vi "Generate.vi"(0 "Snake in":refnum<class "Snake.lvclass">, 1 "Coordinates":T1, 5 "error in (no error)":errorcluster) -> (14 "Snake out":refnum<class "Snake.lvclass">, 19 "error out":errorcluster)   [LabVIEW 2021, in "Snake.lvclass"]
uses:
  Snake.lvclass
  Coordinates.ctl
  Snake.lvclass/Snake.ctl
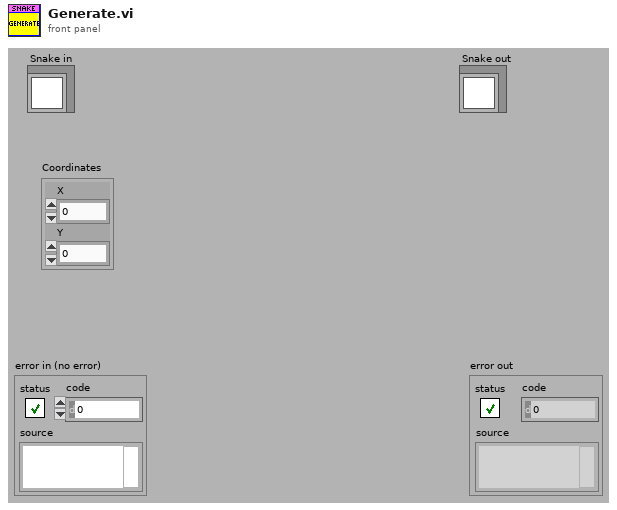
[diagram p1: front panel]
types:
  T1 = typedef "Coordinates.ctl" = cluster{"X":i32, "Y":i32}
  T2 = typedef "Direction.ctl" = enum16{"up", "down", "left", "right"}
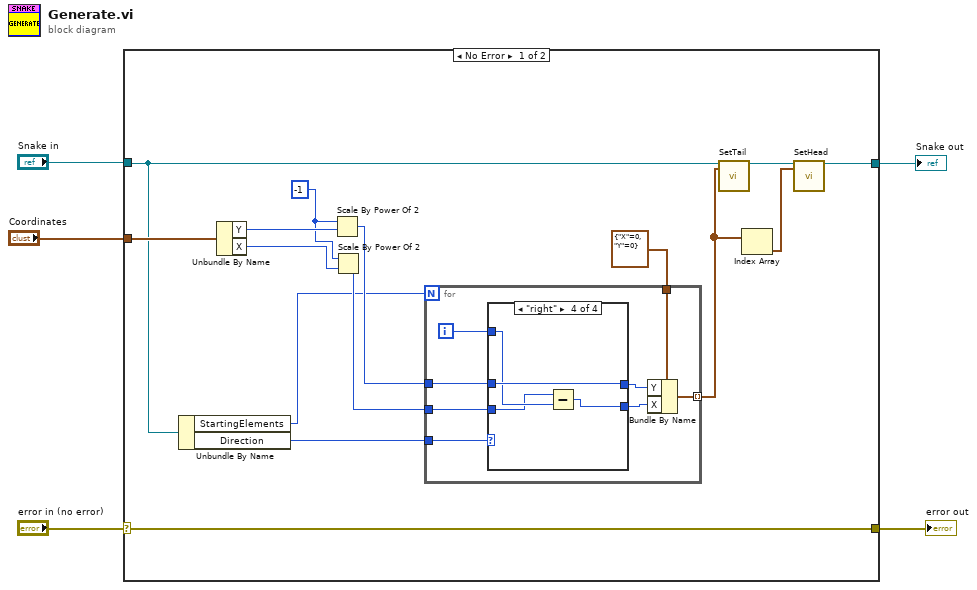
[diagram p0: block diagram]
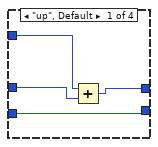
[diagram p2: hidden frame]
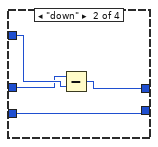
[diagram p3: hidden frame]
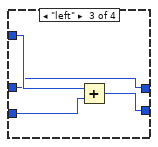
[diagram p4: hidden frame]
diagram:
  n1 = case shown="No Error" "error in (no error)" {
    selector: "error in (no error)" -> [w20 w46]
    tunnel: [w20 w46] -> w4
    tunnel: [w9 w45] -> w2
    tunnel: "Snake in" -> [w11 w45]
    tunnel: "Coordinates" -> [w19 _]
    frame No Error {
      w16 = -1
      n2 = Unbundle By Name(w11) -> ("StartingElements"=w13:i32, "Direction"=w12:T2)
      n3 = Unbundle By Name(w19) -> ("Y"=w17:i32, "X"=w18:i32)
      n4 = Scale By Power Of 2(n=w16, x=w17) -> (x*2^n=w15:i32)
      n5 = Scale By Power Of 2(n=w16, x=w18) -> (x*2^n=w14:i32)
      n6 = for {
        N: w13 -> [_]
        tunnel: w15 -> [w26]
        tunnel: w14 -> [w25]
        tunnel: w12 -> [w27]
        tunnel: [w22] -> w8 mode=indexing
        tunnel: T1 {"X"=0, "Y"=0} ("Coordinates") -> [w21]
        i -> [w28]
        n7 = case shown="\"right\"" w27 {
          tunnel: w28 -> [w31 w35 w40 w43]
          tunnel: w26 -> [w32 w34 w37 w44]
          tunnel: [w30 w33 w37 w44] -> w24
          tunnel: w25 -> [w29 w36 w39 w42]
          tunnel: [w29 w36 w38 w41] -> w23
          frame "up", Default {
            n8 = Add(x=w31, y=w32) -> (x+y=w30:i32)
          }
          frame "down" {
            n9 = Subtract(x=w34, y=w35) -> (x-y=w33:i32)
          }
          frame "left" {
            n10 = Add(x=w40, y=w39) -> (x+y=w38:i32)
          }
          frame "right" {
            n11 = Subtract(x=w42, y=w43) -> (x-y=w41:i32)
          }
        }
        n12 = Bundle By Name(cluster=w21, "Y"=w24, "X"=w23) -> (w22:T1)
      }
      n13 = call-dynamic "SetTail.vi"("object in"=w11, "Tail"=w8) -> ("object out"=w10:refnum<class "Snake.lvclass">)  [unwired: 16 in, 1 out]
      n14 = Index Array(array=w8) -> (element=w7:T1)  [unwired: 1 in]
      n15 = call-dynamic "SetHead.vi"("object in"=w10, "Head"=w7) -> ("object out"=w9:refnum<class "Snake.lvclass">)  [unwired: 16 in, 1 out]
    }
    frame Error {
    }
  }
  "error out" <- w4
  "Snake out" <- w2
